vi "Write to cRIO.vi"(8 "error in (no error)":errorcluster, 11 "Vessel in":refnum<class "Vessel.lvclass">) -> (0 "error out":errorcluster, 3 "Vessel out":refnum<class "Vessel.lvclass">)   [LabVIEW 2014, in "Vessel.lvclass"]
uses:
  Vessel.lvclass
  Vessel.lvclass/Vessel.ctl
  Library/Helping Routines/get_set_point (SubVI).vi
  Supervisor/Supervisor.lvclass
panel:
  in  "Knob":u8(knob)=127 scale=0.0..127.0
  out "Name":string
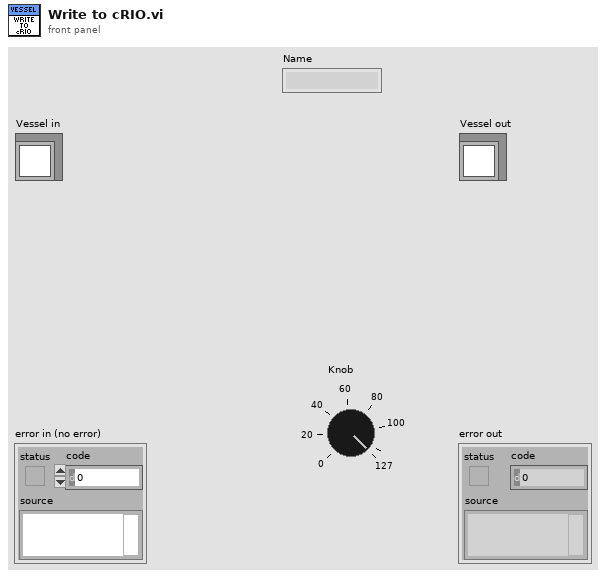
[diagram p1: front panel]
types:
  T1 = cluster{"Measured":cluster{"Eta":dbl[], "Nu":dbl[], "Eta Dot":dbl[], "Nu Dot":dbl[]}, "Estimated":cluster{"Eta":dbl[], "Nu":dbl[], "Eta Dot":dbl[], "Nu Dot":dbl[]}, "Desired":cluster{"Eta":dbl[], "Nu":dbl[], "Eta Dot":dbl[], "Nu Dot":dbl[]}, "Previous Desired":cluster{"Eta":dbl[], "Nu":dbl[], "Eta Dot":dbl[], "Nu Dot":dbl[]}, "tau":dbl[], "Altitude":cluster{"Measured":dbl, "Estimated":dbl, "Desired":dbl, "Previous Desired":dbl, "Approximated":dbl, "grad F":dbl[]}, "rpm":dbl[], "Attitude":cluster{"Theta Measured":dbl[], "Theta Estimated":dbl[], "Omega Measured":dbl[], "Omega Estimated":dbl[], "Gyro Bias":dbl[]}}
  T2 = cluster{"Set Origin":bool, "New WP":bool, "Types of Change":enum16{"Current NED", "Change NED"}, "Make Change":bool, "Optimal Heading":bool, "New SetPoint":cluster{"North":dbl, "East":dbl, "Depth":dbl, "Heading":dbl}, "Update Reference":cluster{"Mode Change":bool, "Current Position":dbl[]}, "Go":bool, "Go heading":bool}
  T3 = cluster{"Pressure +":bool, "Pressure -":bool, "Vacuum +":bool, "Vacuum -":bool}
  T4 = cluster{"In":bool, "Out":bool, "Rotate CW":bool, "Rotate CCW":bool}
  T5 = cluster{"Button 1":bool, "Button 2":bool, "Button 3":bool, "Button 4":bool, "Button 5":bool, "Button 6":bool, "Button 7":bool, "Button 8":bool, "Button 9":bool, "Button 10":bool, "Button 11":bool, "Button 12":bool, "POV Direction":i32}
  T6 = cluster{"Eta":dbl[], "Nu":dbl[], "Eta Dot":dbl[], "Nu Dot":dbl[]}
  T7 = cluster{"Theta Measured":dbl[], "Theta Estimated":dbl[], "Omega Measured":dbl[], "Omega Estimated":dbl[], "Gyro Bias":dbl[]}
  T8 = cluster{"Measured":dbl, "Estimated":dbl, "Desired":dbl, "Previous Desired":dbl, "Approximated":dbl, "grad F":dbl[]}
  T9 = cluster{"HPR":bool, "Sonar 1":bool, "Sonar 2":bool, "Doppler":bool, "Laser":bool, "KRAFT":bool, "Pan/Tilt":bool, "Transponder":bool, "Still Cam":bool, "HD Cam":bool, "UHI Cam":bool}
  T10 = cluster{"Power Switch":bool, "Upper Arm Up":bool, "Upper Arm Down":bool, "Lower Arm Up":bool, "Lower Arm Down":bool, "Arm Left":bool, "Arm Right":bool, "Claw Open":bool, "Claw Close":bool, "Rotate Clockwise":bool, "Rotate Counterclockwise":bool}
  T11 = cluster{"Light 1":bool, "Light 2":bool, "Light 3":bool, "Light 4":bool, "HMI 1":bool, "HMI 2":bool, "Light Intensity 1":i32, "Light Intensity 2":i32, "Light Intensity 3":i8}
  T12 = cluster{"Cam. No.":i32, "Cam Up":bool, "Cam Down":bool, "Cam Left":bool, "Cam Right":bool, "Zoom In":bool, "Zoom Out":bool, "Zoom In 2":bool, "Zoom Out 2":bool}
  T13 = cluster{"Altimeter Active":bool, "Beam select":i8, "Value":cluster{"Measured":dbl, "Estimated":dbl, "Desired":dbl, "Previous Desired":dbl, "Approximated":dbl}}
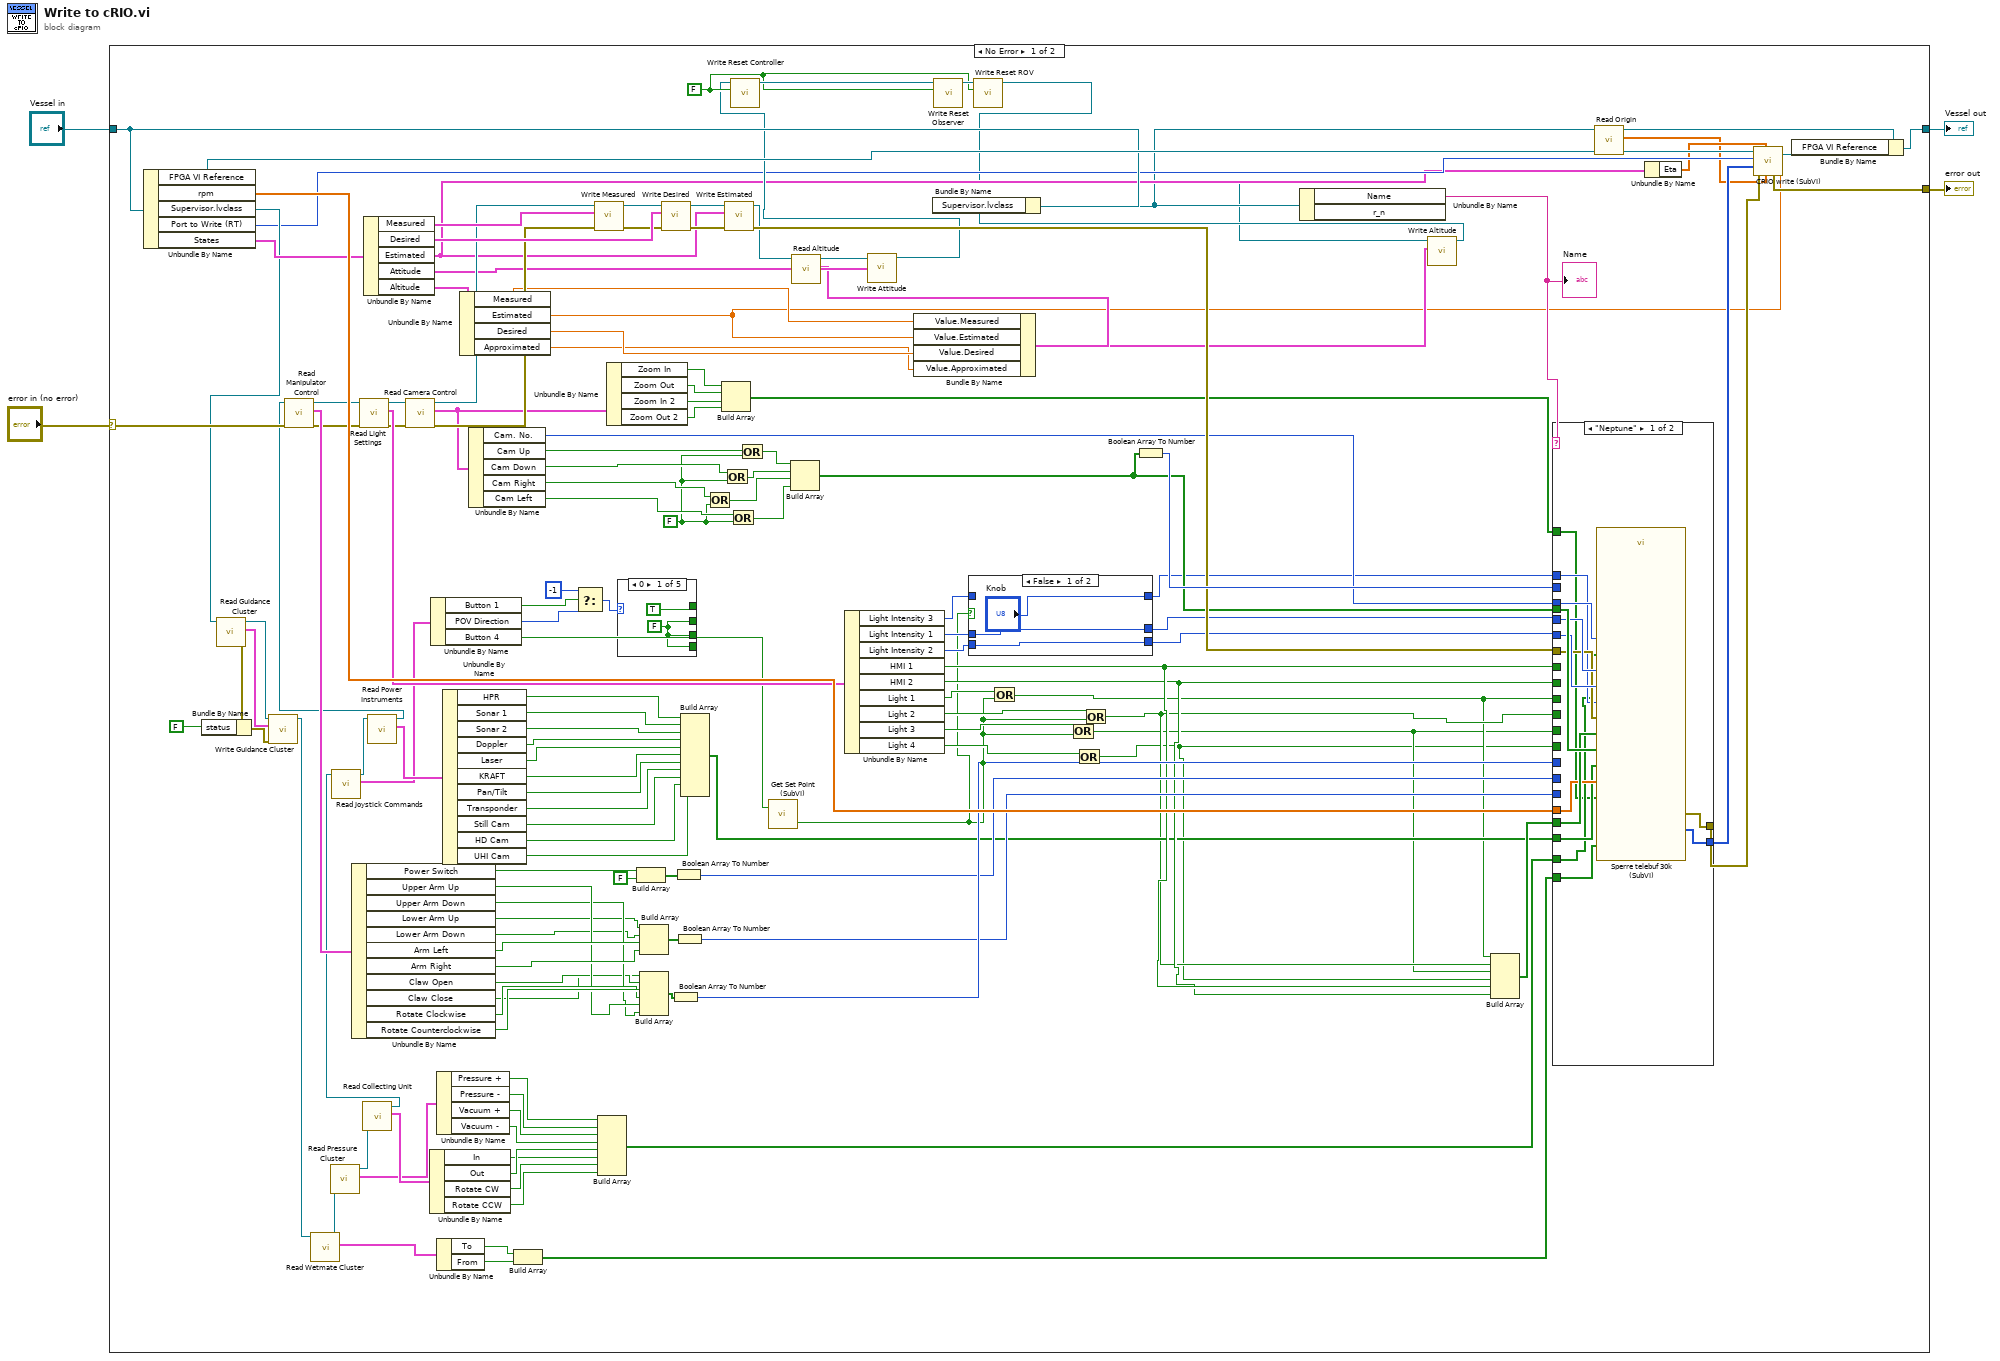
[diagram p0: block diagram]
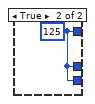
[diagram p2: hidden frame]
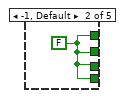
[diagram p3: hidden frame]
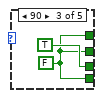
[diagram p4: hidden frame]
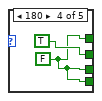
[diagram p5: hidden frame]
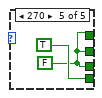
[diagram p6: hidden frame]
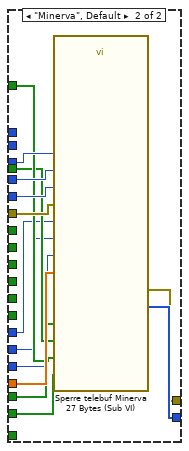
[diagram p7: hidden frame]
diagram:
  n1 = case shown="No Error" "error in (no error)" {
    selector: "error in (no error)" -> [w135 w195]
    tunnel: [w150 w195] -> w3
    tunnel: [w138 w194] -> w1
    tunnel: "Vessel in" -> [w127 w194]
    frame No Error {
      w6 = FALSE ("y")
      w115 = FALSE ("Reset Controller")
      n2 = Unbundle By Name(w127) -> ("FPGA VI Reference"=w151:refnum<k20>, "rpm"=w152:dbl[], "Supervisor.lvclass"=w118:refnum<class "Supervisor.lvclass">, "Port to Write (RT)"=w79:enum8{"1", "2", "3", "4"}, "States"=w132:T1)
      n3 = call-dynamic "Read Guidance Cluster.vi"("Supervisor in"=w118) -> ("error out"=w120:errorcluster, "Guidance Cluster"=w57:T2, "Supervisor out"=w121:refnum<class "Supervisor.lvclass">)  [unwired: 8 in]
      n4 = Bundle By Name(cluster=w120, "status"=FALSE ("Set Origin")) -> (w58:errorcluster)
      n5 = call-dynamic "Write Guidance Cluster.vi"("error in (no error)"=w58, "Guidance Cluster"=w57, "Supervisor in"=w121) -> ("Supervisor out"=w67:refnum<class "Supervisor.lvclass">)  [unwired: 7 in, 1 out]
      n6 = call-dynamic "Read Wetmate Cluster.vi"("Supervisor in"=w67) -> ("Wetmate Cluster"=w65:cluster{"To":bool, "From":bool}, "Supervisor out"=w66:refnum<class "Supervisor.lvclass">)  [unwired: 8 in, 1 out]
      n7 = call-dynamic "Read Pressure Cluster.vi"("Supervisor in"=w66) -> ("Pressure Cluster"=w72:T3, "Supervisor out"=w73:refnum<class "Supervisor.lvclass">)  [unwired: 8 in, 1 out]
      n8 = call-dynamic "Read Collecting Unit.vi"("Supervisor in"=w73) -> ("Collecting Unit"=w97:T4, "Supervisor out"=w55:refnum<class "Supervisor.lvclass">)  [unwired: 8 in, 1 out]
      n9 = call-dynamic "Read Joystick Commands.vi"("Supervisor in"=w55) -> ("Joystick Commands"=w53:T5, "Supervisor out"=w54:refnum<class "Supervisor.lvclass">)  [unwired: 8 in, 1 out]
      n10 = Unbundle By Name(w132) -> ("Measured"=w131:T6, "Desired"=w130:T6, "Estimated"=w60:T6, "Attitude"=w86:T7, "Altitude"=w78:T8)
      n11 = call-dynamic "Read Power Instruments.vi"("Supervisor in"=w54) -> ("Power Instruments"=w109:T9, "Supervisor out"=w110:refnum<class "Supervisor.lvclass">)  [unwired: 8 in, 1 out]
      n12 = call-dynamic "Read Manipulator Control.vi"("error in (no error)"=w135, "Supervisor in"=w110) -> ("error out"=w134:errorcluster, "Manipulator Control"=w146:T10, "Supervisor out"=w137:refnum<class "Supervisor.lvclass">)  [unwired: 7 in]
      n13 = Unbundle By Name(w146) -> ("Power Switch"=w145:bool, "Upper Arm Up"=w25:bool, "Upper Arm Down"=w24:bool, "Lower Arm Up"=w23:bool, "Lower Arm Down"=w22:bool, "Arm Left"=w30:bool, "Arm Right"=w29:bool, "Claw Open"=w21:bool, "Claw Close"=w20:bool, "Rotate Clockwise"=w26:bool, "Rotate Counterclockwise"=w27:bool)
      n14 = call-dynamic "Read Light Settings.vi"("error in (no error)"=w134, "Supervisor in"=w137) -> ("error out"=w133:errorcluster, "Light Settings"=w147:T11, "Supervisor out"=w136:refnum<class "Supervisor.lvclass">)  [unwired: 7 in]
      n15 = call-dynamic "Read Camera Control.vi"("error in (no error)"=w133, "Supervisor in"=w136) -> ("error out"=w126:errorcluster, "Camera Control"=w91:T12, "Supervisor out"=w128:refnum<class "Supervisor.lvclass">)  [unwired: 7 in]
      n16 = Unbundle By Name(w97) -> ("In"=w95:bool, "Out"=w96:bool, "Rotate CW"=w94:bool, "Rotate CCW"=w93:bool)
      n17 = Unbundle By Name(w53) -> ("Button 1"=w35:bool, "POV Direction"=w34:i32, "Button 4"=w52:bool)
      n18 = Unbundle By Name(w72) -> ("Pressure +"=w71:bool, "Pressure -"=w70:bool, "Vacuum +"=w69:bool, "Vacuum -"=w68:bool)
      n19 = Unbundle By Name(w65) -> ("To"=w64:bool, "From"=w63:bool)
      n20 = Unbundle By Name(w109) -> ("HPR"=w108:bool, "Sonar 1"=w107:bool, "Sonar 2"=w106:bool, "Doppler"=w105:bool, "Laser"=w104:bool, "KRAFT"=w103:bool, "Pan/Tilt"=w102:bool, "Transponder"=w101:bool, "Still Cam"=w100:bool, "HD Cam"=w99:bool, "UHI Cam"=w7:bool)
      n21 = Unbundle By Name(w78) -> ("Measured"=w77:dbl, "Estimated"=w5:dbl, "Desired"=w76:dbl, "Approximated"=w74:dbl)
      n22 = Unbundle By Name(w91) -> ("Cam. No."=w56:i32, "Cam Up"=w43:bool, "Cam Down"=w41:bool, "Cam Right"=w39:bool, "Cam Left"=w37:bool)
      n23 = Build Array(w64, w63) -> (w62:bool[])
      n24 = Select(t=-1, s=w35, f=w34) -> (s? t:f=w33:i32)
      n25 = call-dynamic "Write Measured.vi"("error in (no error)"=w126, "Measured"=w131, "Supervisor in"=w128) -> ("error out"=w125:errorcluster, "Supervisor out"=w129:refnum<class "Supervisor.lvclass">)  [unwired: 7 in]
      n26 = Build Array(w71, w70, w69, w68, w96, w95, w94, w93) -> (w92:bool[])
      n27 = Unbundle By Name(w91) -> ("Zoom In"=w90:bool, "Zoom Out"=w89:bool, "Zoom In 2"=w88:bool, "Zoom Out 2"=w87:bool)
      n28 = case shown="0" w33 {
        tunnel: [TRUE w159 w160 w162 w164] -> _
        tunnel: [w157 w159 w160 TRUE w164] -> _
        tunnel: [w157 w159 TRUE w162 w164] -> _
        tunnel: [w157 w159 w160 w162 TRUE] -> _
        frame 0 {
          w157 = FALSE
        }
        frame -1, Default {
          w159 = FALSE
        }
        frame 90 {
          w160 = FALSE
        }
        frame 180 {
          w162 = FALSE
        }
        frame 270 {
          w164 = FALSE
        }
      }
      n29 = Build Array(w145, FALSE ("element")) -> (w144:bool[])
      n30 = Build Array(w23, w22, w30, w29) -> (w28:bool[])
      n31 = Build Array(w20, w21, w27, w26, w25, w24) -> (w143:bool[])
      n32 = call-dynamic "Write Desired.vi"("error in (no error)"=w125, "Desired"=w130, "Supervisor in"=w129) -> ("error out"=w123:errorcluster, "Supervisor out"=w124:refnum<class "Supervisor.lvclass">)  [unwired: 7 in]
      n33 = Boolean Array To Number(Boolean array=w143) -> (number=w142:u32)
      n34 = Boolean Array To Number(Boolean array=w144) -> (number=w141:u32)
      n35 = Boolean Array To Number(Boolean array=w28) -> (number=w140:u32)
      n36 = Build Array(w108, w107, w106, w105, w104, w103, w102, w101, w100, w99, w7) -> (w98:bool[])
      n37 = Or(x=w39, y=w6) -> (x .or. y?=w38:bool)
      n38 = Build Array(w90, w89, w88, w87) -> (w75:bool[])
      n39 = Or(x=w41, y=w6) -> (x .or. y?=w40:bool)
      n40 = call-dynamic "Write Estimated.vi"("error in (no error)"=w123, "Estimated"=w60, "Supervisor in"=w124) -> ("error out"=w122:errorcluster, "Supervisor out"=w83:refnum<class "Supervisor.lvclass">)  [unwired: 7 in]
      n41 = Or(x=w37, y=w6) -> (x .or. y?=w36:bool)
      n42 = Or(x=w43, y=w6) -> (x .or. y?=w42:bool)
      n43 = call-poly "Get Set Point (SubVI).vi"("auto set  in"=w52) -> ("auto set"=w8:bool)  [unwired: 1 in, 1 out]
      n44 = Build Array(w42, w40, w38, w36) -> (w114:bool[])
      n45 = call-dynamic "Read Altitude.vi"("Supervisor in"=w83) -> ("Altitude"=w84:T13, "Supervisor out"=w82:refnum<class "Supervisor.lvclass">)  [unwired: 8 in, 1 out]
      n46 = Unbundle By Name(w147) -> ("Light Intensity 3"=w13:i8, "Light Intensity 1"=w11:i32, "Light Intensity 2"=w9:i32, "HMI 1"=w113:bool, "HMI 2"=w112:bool, "Light 1"=w51:bool, "Light 2"=w50:bool, "Light 3"=w47:bool, "Light 4"=w45:bool)
      n47 = call-dynamic "Write Attitude.vi"("Attitude"=w86, "Supervisor in"=w82) -> ("Supervisor out"=w85:refnum<class "Supervisor.lvclass">)  [unwired: 8 in, 1 out]
      n48 = call-dynamic "Write Reset Controller.vi"("Reset Controller"=w115, "Supervisor in"=w85) -> ("Supervisor out"=w117:refnum<class "Supervisor.lvclass">)  [unwired: 8 in, 1 out]
      n49 = Bundle By Name(cluster=w84, "Value.Measured"=w77, "Value.Estimated"=w5, "Value.Desired"=w76, "Value.Approximated"=w74) -> (w81:T13)
      n50 = call-dynamic "Write Reset Observer.vi"("Reset Observer"=w115, "Supervisor in"=w117) -> ("Supervisor out"=w116:refnum<class "Supervisor.lvclass">)  [unwired: 8 in, 1 out]
      n51 = case shown="False" w8 {
        tunnel: ["Knob" w156] -> w14
        tunnel: w13 -> [_ _]
        tunnel: [w155 w156] -> w12
        tunnel: w11 -> [w155 _]
        tunnel: [w154 w156] -> w10
        tunnel: w9 -> [w154 _]
        frame False {
        }
        frame True {
          w156 = i8 125 ("Light Intensity 3")
        }
      }
      n52 = call-dynamic "Write Reset ROV.vi"("Reset ROV"=w115, "Supervisor in"=w116) -> ("Supervisor out"=w16:refnum<class "Supervisor.lvclass">)  [unwired: 8 in, 1 out]
      n53 = Or(x=w51, y=w8) -> (x .or. y?=w48:bool)
      n54 = Or(x=w47, y=w8) -> (x .or. y?=w46:bool)
      n55 = Or(x=w45, y=w8) -> (x .or. y?=w44:bool)
      n56 = Or(x=w50, y=w8) -> (x .or. y?=w49:bool)
      n57 = Boolean Array To Number(Boolean array=w114) -> (number=w148:u32)
      n58 = call-dynamic "Write Altitude.vi"("Altitude"=w81, "Supervisor in"=w16) -> ("Supervisor out"=w80:refnum<class "Supervisor.lvclass">)  [unwired: 8 in, 1 out]
      n59 = Bundle By Name(cluster=w127, "Supervisor.lvclass"=w80) -> (w18:refnum<class "Vessel.lvclass">)
      n60 = Unbundle By Name(w18) -> ("Name"=w15:string)  [unwired: 1 out]
      "Name" <- w15
      n61 = Build Array(w48, w49, w46, w44, w113, w112) -> (w111:bool[])
      n62 = case shown="\"Neptune\"" w15 {
        tunnel: w152 -> [w171 w188]
        tunnel: [w179 w192] -> w61
        tunnel: [w178 w191] -> w149
        tunnel: w113 -> [_ _]
        tunnel: w112 -> [_ _]
        tunnel: w48 -> [_ _]
        tunnel: w49 -> [_ _]
        tunnel: w46 -> [_ _]
        tunnel: w44 -> [_ _]
        tunnel: w12 -> [w175 w190]
        tunnel: w10 -> [w174 w189]
        tunnel: w148 -> [_ _]
        tunnel: w56 -> [w173 w193]
        tunnel: w142 -> [_ w183]
        tunnel: w141 -> [_ w182]
        tunnel: w140 -> [_ w181]
        tunnel: w122 -> [w172 w186]
        tunnel: w114 -> [w177 w184]
        tunnel: w111 -> [w176 w187]
        tunnel: w98 -> [w170 w180]
        tunnel: w14 -> [w169 _]
        tunnel: w92 -> [w168 _]
        tunnel: w75 -> [w167 w185]
        tunnel: w62 -> [w166 _]
        frame "Neptune" {
          n63 = call "Sperre telebuf 30k (SubVI).vi"("Thruster rpms"=w171, "pan tilt"=w177, "Lights/HMI"=w176, "Wetmate"=w166, "error in"=w172, "dim 1"=w175, "Power Instruments"=w170, "dim 2"=w174, "Collecting Unit"=w168, "dim 34"=w169, "Zoom 1-2"=w167, "cam no"=w173) -> ("telebuf out"=w179:u8[], "error IO"=w178:errorcluster)  [unwired: 6 in]
        }
        frame "Minerva", Default {
          n64 = call "Sperre telebuf Minerva 27 Bytes (Sub VI).vi"("Thruster rpms"=w188, "manip1"=w183, "manip2"=w182, "manip3"=w181, "Pan_tilt"=w184, "error in"=w186, "dim 1+2"=w190, "Lights_HMI"=w187, "dim 3+4"=w189, "Zoom"=w185, "Power"=w180, "camera"=w193) -> ("telebuf"=w192:u8[], "error IO"=w191:errorcluster)  [unwired: 6 in]
        }
      }
      n65 = call-dynamic "Read Origin.vi"("Vessel in"=w18) -> ("Origin"=w19:dbl[], "Vessel out"=w17:refnum<class "Vessel.lvclass">)  [unwired: 8 in, 1 out]
      n66 = Unbundle By Name(w60) -> ("Eta"=w59:dbl[])
      n67 = call "CRIO write (SubVI).vi"("Altitude Est"=w5, "CO_NED"=w19, "States"=w59, "error IO"=w149, "Array"=w61, "Port to Write (RT)"=w79, "FPGA VI Reference In"=w151) -> ("error out"=w150:errorcluster, "FPGA VI Reference Out"=w139:refnum<k20>)  [unwired: 3 in]
      n68 = Bundle By Name(cluster=w17, "FPGA VI Reference"=w139) -> (w138:refnum<class "Vessel.lvclass">)
    }
    frame Error {
    }
  }
  "error out" <- w3
  "Vessel out" <- w1
